vi "path_empty_check.vi"(8 "error in":errorcluster, 11 "path_Input":path) -> (0 "error out":errorcluster, 2 "bo_exist":bool, 3 "bo_Empty":bool)   [LabVIEW 2026]
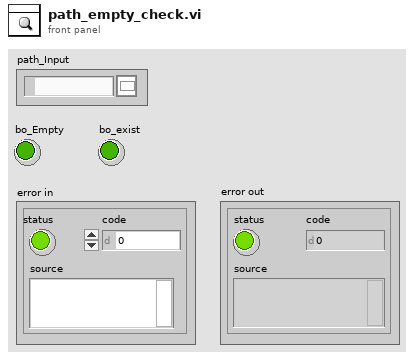
[diagram p1: front panel]
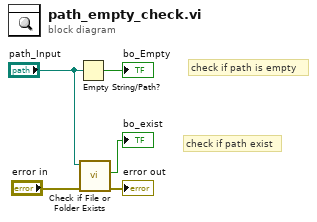
[diagram p0: block diagram]
diagram:
  # "check if path exist"
  # "check if path is empty"
  n1 = Empty String/Path?(string/path="path_Input") -> (empty?=→"bo_Empty":bool)
  n2 = call <vilib>:"Check if File or Folder Exists.vi"("error in (no error)"="error in", "path"="path_Input") -> ("error out"=→"error out":errorcluster, "file or folder exists?"=→"bo_exist":bool)  [unwired: 7 in, 1 out]
